vi "Remove Child Unified Actor.vi"(7 "Actor in":refnum<class "Actor.lvclass">, 10 "Unified Actor Alias":string) -> (5 "Actor out":refnum<class "Actor.lvclass">)   [LabVIEW 2020, in "jettl.lvlib"]
uses:
  jettl.lvlib
  Actor/Actor.lvclass
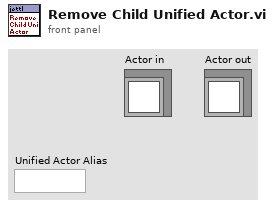
[diagram p1: front panel]
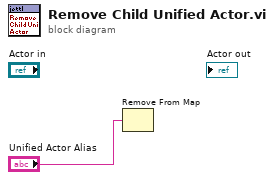
[diagram p0: block diagram]
diagram:
  n1 = Remove From Map(10:"Unified Actor Alias") -> (11:w1:map{string, i32})  [unwired: 3 out]
